vi "Manual Test.vi"() -> ()   [LabVIEW 2016]
uses:
  <vilib>/Platform/TimedLoop/XDataNode/timing_clust.ctl
  <vilib>/Platform/TimedLoop/XDataNode/nitl_modes.ctl
  <vilib>/Platform/TimedLoop/XDataNode/wakeup.ctl
  <vilib>/platform/TimedLoop/XDataNode/XDataNode.xnode
  Assert API Components/Assert API Components.lvlib
  <vilib>/Platform/TimedLoop/XDataNode/XDNodeRunTimeDep.lvlib
panel:
  in  "Period":i64=10000
  in  "stop":bool
  in  "Data Type":string="strng"
  in  "Comment":string="blah blah blah"
  in  "Assert VI UID":i32
  in  "Evaluation String":string
  in  "Assert Build Timestamp":timestamp
  in  "Last Update":timestamp
  in  "Assert Builder User Name":string
  in  "Failure Action":string="None"
  in  "Top Level VI Name":string
  in  "Calling VI Name":string="blahs caller"
  in  "Assert VI Name":string="blah"
  in  "Status":bool
  in  "Data Value":variant
  in  "Assert Name":string="test"
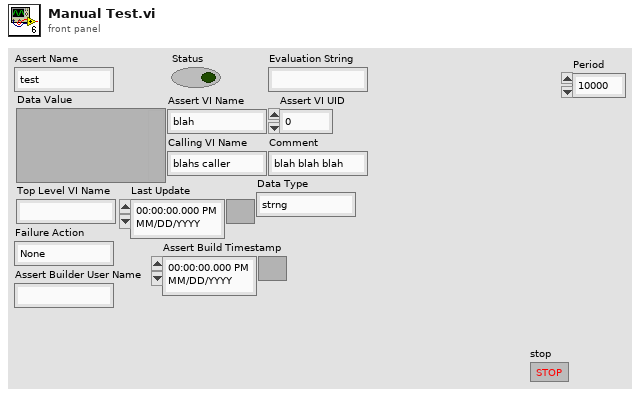
[diagram p1: front panel]
types:
  T1 = typedef "XDNodeRunTimeDep.lvlib/timing_clust.ctl" = cluster{"Expected End [f-1]":u64, "Actual End [f-1]":u64, "Finished Late? [f-1]":bool, "Expected End [i-1]":u64, "Actual End [i-1]":u64, "Finished Late? [i-1]":bool, "Expected Start [i]":u64, "Actual Start [i]":u64, "Expected Start [f]":u64, "Actual Start [f]":u64, "Source Name":string, "Structure Name":string, "Period":i64, "Deadline":i64, "Offset":i64, "Start":i64, "Priority":i32, "Timeout":i32, "Mode":T2, "Wakeup Reason":T3, "Error":errorcluster, "Source Type":string, "Secondary Source Type":string, "Global End Time":u64, "Global Start Time":u64, "Frame Duration":u64, "Iteration Duration":u64, "Assigned CPU":i32, "I/O Scan Engine Mode":u32}
  T2 = typedef "XDNodeRunTimeDep.lvlib/nitl_modes.ctl" = enum32{"No Change", "Process missed periods, maintain original phase", "Discard missed periods, maintain original phase", "Process missed periods, ignore original phase", "Discard missed periods, ignore original phase"}
  T3 = typedef "XDNodeRunTimeDep.lvlib/wakeup.ctl" = enum32{"Normal", "Aborted", "Asynchronous wakeup", "Timing source error", "Timed loop error", "Timeout"}
  T4 = cluster{"This VI":refnum<vi>, "Calling VI's Reference":refnum<vi>}
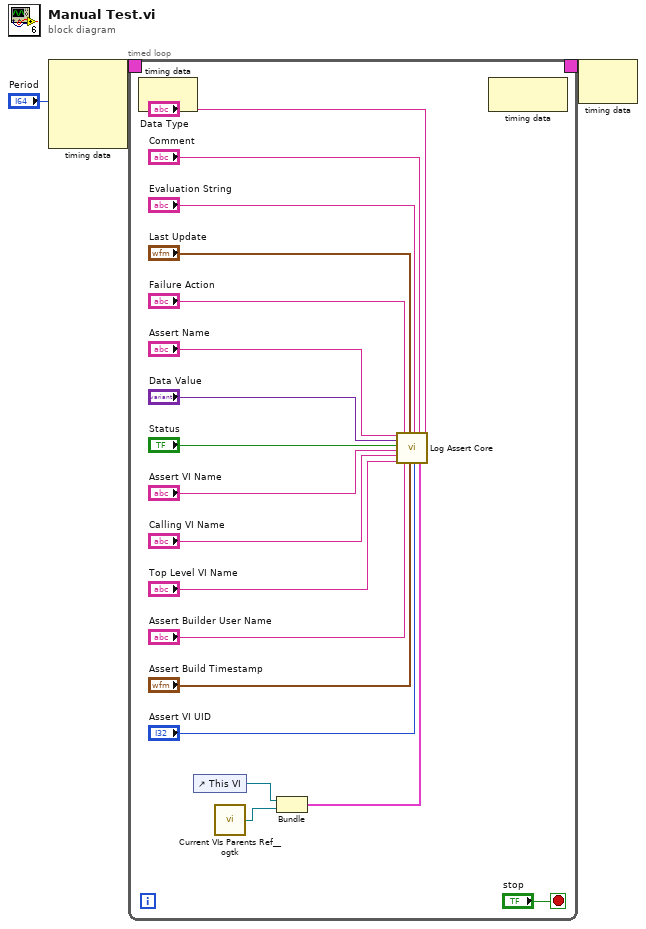
[diagram p0: block diagram]
diagram:
  n1 = node-c288("Period") -> (w3:T1)  [unwired: 3 in]
  n2 = timed-loop {
    timing: w3 -> [_]
    timing-out: [_] -> w2
    stop <- "stop" stop-if-true
    n3 = node-c288() -> ()  [unwired: 1 in, 1 out]
    n4 = control-ref of="This VI"() -> (w6:refnum<vi>)
    n5 = call <userlib>:"Current VIs Parents Ref__ogtk.vi"() -> ("Calling VI's Reference"=w5:refnum<vi>)  [unwired: 2 in]
    n6 = Bundle("This VI"=w6, "Calling VI's Reference"=w5) -> (w4:T4)  [unwired: 1 in]
    n7 = call "Log Assert Core.vi"("Assert Name"="Assert Name", "Data Value"="Data Value", "Status"="Status", "Assert VI Name"="Assert VI Name", "Calling VI Name"="Calling VI Name", "Top Level VI Name"="Top Level VI Name", "Failure Action"="Failure Action", "Assert Builder User Name"="Assert Builder User Name", "Last Update"="Last Update", "Assert Build Timestamp"="Assert Build Timestamp", "Evaluation String"="Evaluation String", "Assert VI UID"="Assert VI UID", "Comment"="Comment", "VI References"=w4, "Data Type"="Data Type") -> ()  [unwired: 5 in]
    n8 = node-c288() -> ()  [unwired: 1 in, 1 out]
  }
  n9 = node-c288(w2) -> ()  [unwired: 1 out]
